vi "RAMP_save_path_definition_sCMOS_movie.vi"(5 "error in":errorcluster, 6 "Sample name":string, 8 "Path to the saving folder":path) -> (0 "error out":errorcluster, 3 "Movie path":path)   [LabVIEW 2015]
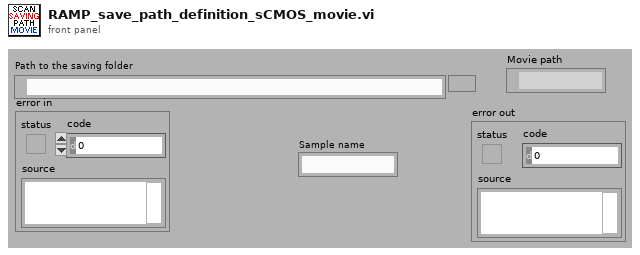
[diagram p1: front panel]
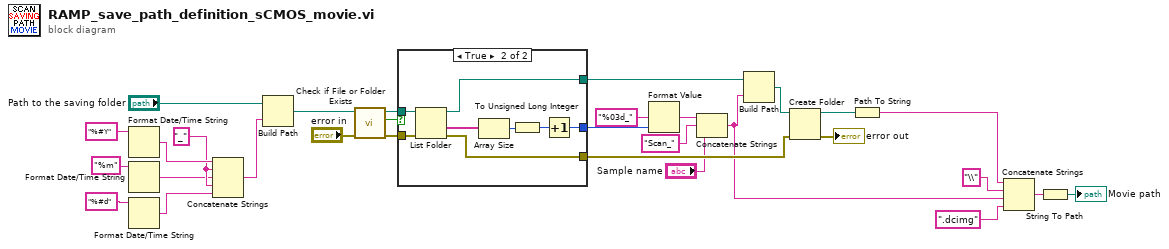
[diagram p0: block diagram]
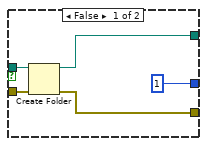
[diagram p2: hidden frame]
diagram:
  w28 = "_" ("string")
  n1 = Format Date/Time String(time format string (%c)="%#Y") -> (date/time string=w29:string)  [unwired: 2 in]
  n2 = Format Date/Time String(time format string (%c)="%m") -> (date/time string=w25:string)  [unwired: 2 in]
  n3 = Format Date/Time String(time format string (%c)="%#d") -> (date/time string=w24:string)  [unwired: 2 in]
  n4 = Concatenate Strings(w29, w28, w25, w28, w24) -> (w22:string)
  n5 = Build Path(base path="Path to the saving folder", name or relative path=w22) -> (appended path=w21:path)
  n6 = call <vilib>:"Check if File or Folder Exists.vi"("error in (no error)"="error in", "path"=w21) -> ("error out"=w6:errorcluster, "file or folder exists?"=w7:bool, "dup path"=w8:path)  [unwired: 7 in]
  n7 = case shown="True" w7 {
    tunnel: w6 -> [w35 w43]
    tunnel: w8 -> [w34 w42]
    tunnel: [w33 w41] -> w12
    tunnel: [w32 w40] -> w19
    tunnel: [u32 1 w37] -> w16
    frame False {
      n8 = Create Folder(path (use dialog)=w34, error in=w35) -> (created path=w32:path, error out=w33:errorcluster)  [unwired: 1 in, 1 out]
    }
    frame True {
      n9 = List Folder(path=w42, error in=w43) -> (path out=w40:path, folder names=w38:string[], error out=w41:errorcluster)  [unwired: 2 in, 1 out]
      n10 = Array Size(array=w38) -> (size(s)=w39:i32)
      n11 = To Unsigned Long Integer(number=w39) -> (unsigned 32bit integer=w36:u32)
      n12 = Increment(x=w36) -> (x+1=w37:u32)
    }
  }
  n13 = Format Value(format string="%03d_" ("string (\"\")"), value (0)=w16) -> (output string=w15:string)  [unwired: 1 in]
  n14 = Concatenate Strings(w15, "Scan_" ("string"), "Sample name") -> (w1:string)
  n15 = Build Path(base path=w19, name or relative path=w1) -> (appended path=w13:path)
  n16 = Create Folder(path (use dialog)=w13, error in=w12) -> (created path=w11:path, error out=→"error out":errorcluster)  [unwired: 1 in, 1 out]
  n17 = Path To String(path=w11) -> (string=w9:string)
  n18 = Concatenate Strings(w9, "\\" ("string"), w1, ".dcimg" ("string")) -> (w4:string)
  n19 = String To Path(string=w4) -> (path=→"Movie path":path)
